vi "IntakeTeleop.vi"(5 "CmdIntakeCoral":bool, 7 "CmdIntakeAlgae":bool, 9 "CmdIntakeCancel":bool, 10 "CmdIntakeDepositAlgae":bool, 11 "CmdIntakeDepositCoral":bool) -> ()   [LabVIEW 2023]
doc: "Makes sure the actual position of the arm is within 5 degrees of the setpoint/target"
uses:
  <vilib>/Rock Robotics/WPI/ThirdParty/JAS_Junk/TrajLib/Trajectory_Library.lvlib
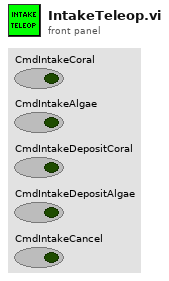
[diagram p1: front panel]
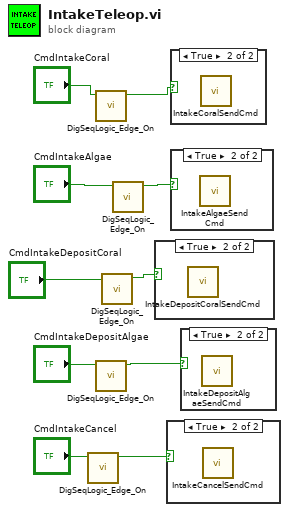
[diagram p0: block diagram]
diagram:
  n1 = call <vilib>:"DigSeqLogic_Edge_On.vi"("Input"="CmdIntakeCancel") -> ("On Edge"=w9:bool)  [unwired: 10 in]
  n2 = call <vilib>:"DigSeqLogic_Edge_On.vi"("Input"="CmdIntakeCoral") -> ("On Edge"=w1:bool)  [unwired: 10 in]
  n3 = call <vilib>:"DigSeqLogic_Edge_On.vi"("Input"="CmdIntakeDepositAlgae") -> ("On Edge"=w7:bool)  [unwired: 10 in]
  n4 = call <vilib>:"DigSeqLogic_Edge_On.vi"("Input"="CmdIntakeDepositCoral") -> ("On Edge"=w10:bool)  [unwired: 10 in]
  n5 = call <vilib>:"DigSeqLogic_Edge_On.vi"("Input"="CmdIntakeAlgae") -> ("On Edge"=w8:bool)  [unwired: 10 in]
  n6 = case shown="True" w10 {
    frame False {
    }
    frame True {
      n7 = call "IntakeDepositCoralSendCmd.vi"() -> ()  [unwired: 11 in, 1 out]
    }
  }
  n8 = case shown="True" w9 {
    frame False {
    }
    frame True {
      n9 = call "IntakeCancelSendCmd.vi"() -> ()  [unwired: 11 in, 1 out]
    }
  }
  n10 = case shown="True" w1 {
    frame False {
    }
    frame True {
      n11 = call "IntakeCoralSendCmd.vi"() -> ()  [unwired: 11 in, 1 out]
    }
  }
  n12 = case shown="True" w8 {
    frame False {
    }
    frame True {
      n13 = call "IntakeAlgaeSendCmd.vi"() -> ()  [unwired: 11 in, 1 out]
    }
  }
  n14 = case shown="True" w7 {
    frame False {
    }
    frame True {
      n15 = call "IntakeDepositAlgaeSendCmd.vi"() -> ()  [unwired: 11 in, 1 out]
    }
  }
